vi "MSScript set_layout.vi"(4 "instr param table":refnum<vi>, 6 "user param table":refnum<vi>, 8 "error in (no error)":errorcluster, 10 "dialogue_top_spl":refnum<vi>, 11 "Parameter Tab":refnum<vi>) -> (0 "error out":errorcluster)   [LabVIEW 2018]
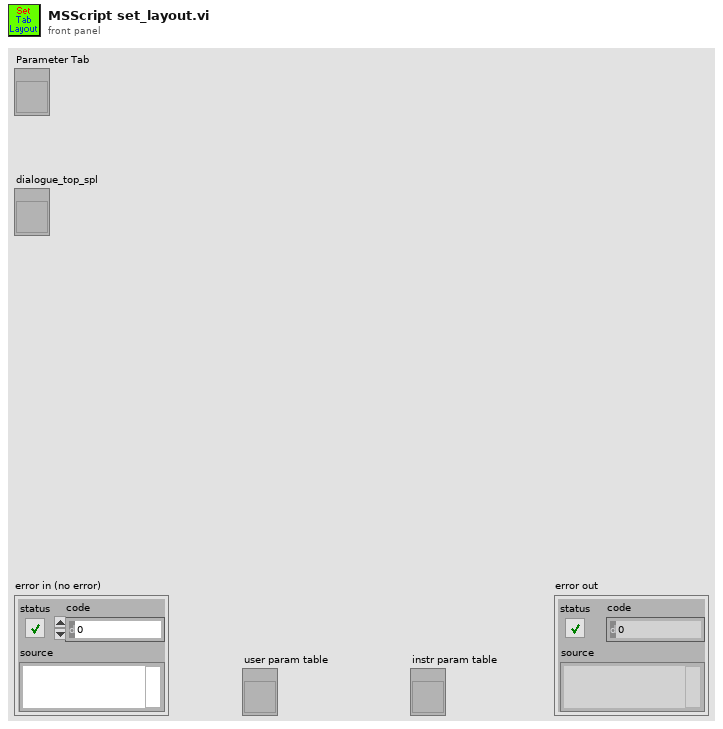
[diagram p1: front panel]
types:
  T1 = enum16{"No Scaling", "Scale All Objects", "Scale Single Object"}
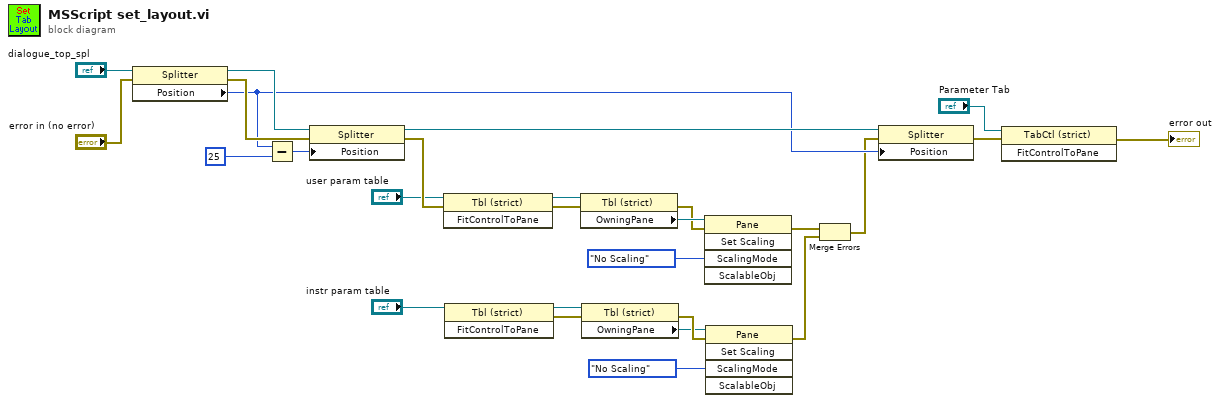
[diagram p0: block diagram]
diagram:
  n1 = property class="Splitter"(reference="dialogue_top_spl", error in="error in (no error)") -> (reference out=w17:refnum<vi>, error out=w18:errorcluster, "Position"=w16:i32)
  n2 = Subtract(x=w16, y=u32 25) -> (x-y=w21:u32)
  n3 = property class="Splitter"(reference=w17, error in=w18, "Position"=w21) -> (reference out=w19:refnum<vi>, error out=w20:errorcluster)
  n4 = invoke class="Tbl (strict)" method="FitControlToPane"(reference="user param table", error in=w20) -> (reference out=w23:refnum<vi>, error out=w22:errorcluster)  [unwired: 1 in, 1 out]
  n5 = invoke class="Tbl (strict)" method="FitControlToPane"(reference="instr param table") -> (reference out=w9:refnum<vi>, error out=w10:errorcluster)  [unwired: 2 in, 1 out]
  n6 = property class="Tbl (strict)"(reference=w23, error in=w22) -> (error out=w24:errorcluster, "OwningPane"=w26:refnum<vi>)  [unwired: 1 out]
  n7 = property class="Tbl (strict)"(reference=w9, error in=w10) -> (error out=w8:errorcluster, "OwningPane"=w6:refnum<vi>)  [unwired: 1 out]
  n8 = invoke class="Pane" method="Set Scaling"(reference=w26, error in=w24, "ScalingMode"=T1."No Scaling" ("Scaling Mode")) -> (error out=w4:errorcluster)  [unwired: 2 in, 4 out]
  n9 = invoke class="Pane" method="Set Scaling"(reference=w6, error in=w8, "ScalingMode"=T1."No Scaling" ("Scaling Mode")) -> (error out=w3:errorcluster)  [unwired: 2 in, 4 out]
  n10 = Merge Errors(w4, w3) -> (w2:errorcluster)
  n11 = property class="Splitter"(reference=w19, error in=w2, "Position"=w16) -> (error out=w11:errorcluster)  [unwired: 1 out]
  n12 = invoke class="TabCtl (strict)" method="FitControlToPane"(reference="Parameter Tab", error in=w11) -> (error out=→"error out":errorcluster)  [unwired: 1 in, 2 out]
